vi "Get status DSP402.vi"(4 "error in (no error)":errorcluster, 6 "Fallback mode":T1 items=["Undefined"=0, "Profile Position Mode"=1, "Velocity Mode"=2, "Profile Velocity Mode"=3, "Torque Profile Mode"=4, "Homing Mode"=6, "Interpolated Position Mode"=7], 7 "DSP402 in":refnum<class "DSP402.lvclass">) -> (0 "error out":errorcluster, 3 "DSP402 out":refnum<class "DSP402.lvclass">)   [LabVIEW 2017, in "canopen.lvlib" / "DSP402.lvclass"]
uses:
  DSP402.lvclass
  DriveMode.ctl
  CANopen/Multiplexor.ctl
  DSP402.lvclass/DSP402.ctl
  CANopen/CANopen.lvclass
panel:
  out "Dummy":variant
  out "Status":u16
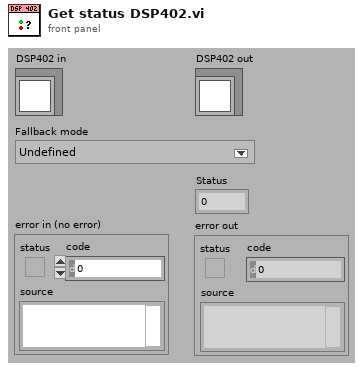
[diagram p1: front panel]
types:
  T1 = typedef "canopen.lvlib/DSP402.lvclass/DriveMode.ctl" = i8
  T2 = typedef "canopen.lvlib/CANopen.lvclass/Multiplexor.ctl" = cluster{"Index":u16, "Sub-index":u8}
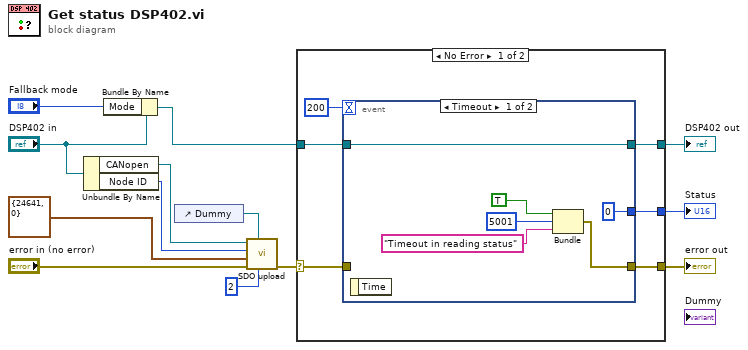
[diagram p0: block diagram]
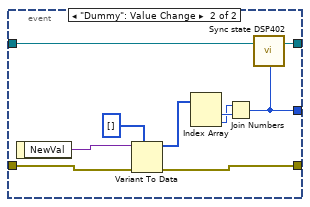
[diagram p2: hidden frame]
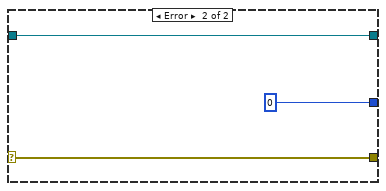
[diagram p3: hidden frame]
diagram:
  n1 = Unbundle By Name("DSP402 in") -> ("CANopen"=w12:refnum<class "CANopen.lvclass">, "Node ID"=w8:u8)
  n2 = Bundle By Name(cluster="DSP402 in", "Mode"="Fallback mode") -> (w1:refnum<class "DSP402.lvclass">)
  n3 = control-ref of="Dummy"() -> (w7:refnum<vi>)
  n4 = call "SDO upload.vi"("Size"=u8 2, "Destination"=w7, "error in (no error)"="error in (no error)", "Multiplexor"=T2 {"Index"=24641, "Sub-index"=0}, "Node ID"=w8, "CANopen in"=w12) -> ("error out"=w6:errorcluster)  [unwired: 3 out]
  n5 = case shown="No Error" w6 {
    selector: w6 -> [w18 w36]
    tunnel: [w15 w38] -> w13
    tunnel: w1 -> [w16 w38]
    tunnel: [w17 w36] -> w5
    tunnel: [w14 u16 0 ("Status")] -> w4
    frame No Error {
      n6 = event shown="[0] Timeout" {
        selector: _ -> [_ _]
        dyn-events: _ -> [_ _]
        timeout: 200 -> [_ _]
        tunnel: w18 -> [_ w35]
        tunnel: [w21 w32] -> w17
        tunnel: w16 -> [w25 w31]
        tunnel: [w25 w33] -> w15
        tunnel: [u16 0 ("Status") w26] -> w14
        event Timeout {
          n7 = event-data() -> ()  [unwired: 2 out]
          n8 = Bundle("status"=TRUE, "code"=5001, "source"="Timeout in reading status") -> (w21:errorcluster)  [unwired: 1 out]
        }
        event "Dummy": Value Change {
          n9 = event-data() -> ("NewVal"=w34:variant)  [unwired: 1 out]
          n10 = Variant To Data(error in=w35, type=u8[] [] ("Data"), Variant=w34) -> (data=w29:u8[], error out=w32:errorcluster)
          n11 = Index Array(array=w29) -> (element #1=w28:u8, element #2=w27:u8)  [unwired: 2 in]
          n12 = Join Numbers(hi=w27, lo=w28) -> ((hi.lo)=w26:u16)
          n13 = call "Sync state DSP402.vi"("Status"=w26, "DSP402 in"=w31) -> ("DSP402 out"=w33:refnum<class "DSP402.lvclass">)  [unwired: 1 out]
        }
      }
    }
    frame Error {
    }
  }
  "error out" <- w5
  "DSP402 out" <- w13
  "Status" <- w4
